vi "Write CSV File_1D.vi"(7 "delimiter (,)":string=",", 8 "error in (no error)":errorcluster, 9 "append to file? (new file)":bool, 10 "1D array":string[](array[string]), 11 "file path in":path) -> (0 "error out":errorcluster, 3 "file path out":path)   [LabVIEW 2012, in "Robust CSV.lvlib"]
doc: "Write a single CSV record to CSV file. The CSV file is formatted in accordance with RFC-4180 (see http://tools.ietf.org/html/rfc4180). \n\nA custom delimiter character can be specified. Default is a comma.\n\nSetting \"append to file?\" to true will append a single record to the end of an existing file. Setting \"append to file?\" to false will overwrite an existing file. In both cases, if the file is not found, a new file will be created.\n\nRev 0.0 2014-02-20 Ryan Porter\n- First Draft\n\nRev 0.1 2014-10-30 Ryan Porter\n- Removed \"Convert EOL\" option from write to file."
uses:
  Robust CSV.lvlib
panel:
  # "Write CSV File_1D.vi\n\nWrite a single CSV record to CSV file. The CSV file is formatted in accordance with RFC-4180 (see http://tools.ietf.org/html/rfc4180). \n\nA custom delimiter character can be specified. Default is a comma.\n\nSetting \"append to file?\" to true will append a single record to the end of an existing file. Setting \"append to file?\" to false will overwrite an existing file. In both cases, if the file is not found, a new file will be created."
  # "License: BSD (2-Clause) - http://opensource.org/licenses/BSD-2-Clause \n\nCopyright (c) 2014, Ryan Porter\nAll rights reserved."
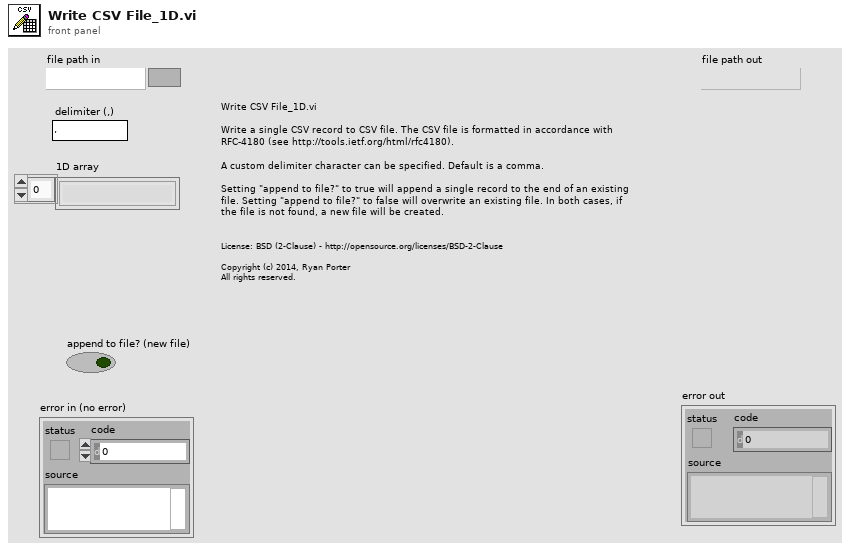
[diagram p1: front panel]
types:
  T1 = enum16{"open", "replace", "create", "open or create", "replace or create", "replace or create with confirmation"}
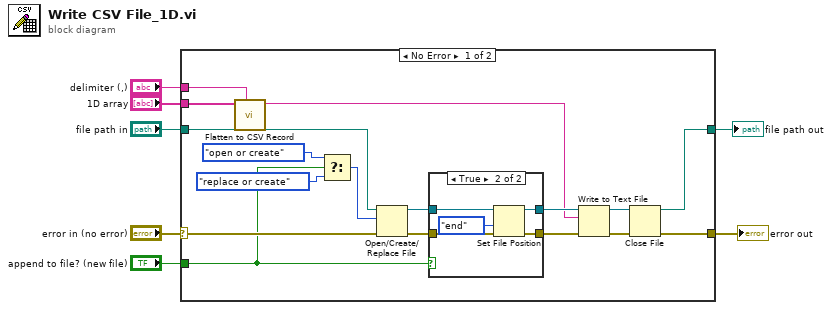
[diagram p0: block diagram]
diagram:
  n1 = case shown="No Error" "error in (no error)" {
    selector: "error in (no error)" -> [w24 w33]
    tunnel: "1D array" -> [w10 _]
    tunnel: "delimiter (,)" -> [w9 _]
    tunnel: [w13 w33] -> w4
    tunnel: "file path in" -> [w23 w32]
    tunnel: "append to file? (new file)" -> [w15 _]
    tunnel: [w11 w32] -> w1
    frame No Error {
      n2 = call "Flatten to CSV Record.vi"("delimiter (,)"=w9, "row of strings"=w10) -> ("CSV record"=w8:string)  [unwired: 1 in, 8 out]
      n3 = Select(t=T1."open or create" ("operation (0:open)"), s=w15, f=T1."replace or create" ("operation (0:open)")) -> (s? t:f=w20:T1)
      n4 = Open/Create/Replace File(file path (use dialog)=w23, error in=w24, operation (0:open)=w20) -> (refnum out=w19:refnum<file>, error out=w18:errorcluster)  [unwired: 4 out]
      n5 = case shown="True" w15 {
        tunnel: w19 -> [w26 w31]
        tunnel: w18 -> [w25 w30]
        tunnel: [w25 w28] -> w17
        tunnel: [w26 w27] -> w16
        frame False {
        }
        frame True {
          n6 = Set File Position(refnum=w31, from (0:start)=enum16{"start", "end", "current"}."end", error in=w30) -> (refnum out=w27:refnum<file>, error out=w28:errorcluster)  [unwired: 1 out]
        }
      }
      n7 = Write to Text File(file (use dialog)=w16, text=w8, error in=w17) -> (refnum out=w12:refnum<file>, error out=w14:errorcluster)  [unwired: 2 out]
      n8 = Close File(refnum=w12, error in=w14) -> (path=w11:path, error out=w13:errorcluster)
    }
    frame Error {
    }
  }
  "error out" <- w4
  "file path out" <- w1
